vi "Configure Math Basic.vi"(0 "VISA resource name":refnum<visa-resource-name>, 1 "GX/GP START/STOP Key Action (1: Start/Stop)":u16(ring)=1 items=["Off", "Start/Stop", "Reset + Start/Stop"], 5 "Value On Error (0: +Over)":u16(ring) items=["+Over", "-Over"], 7 "Overflow Value 1 (1: Skip)":u16(ring)=1 items=["Error", "Skip", "Limit"], 9 "Overflow Value 2 (0: Over)":u16(ring) items=["Over", "Skip"], 11 "error in (no error)":errorcluster, 12 "GM START Key Action (0: Not Change)":u16(ring) items=["Not Change", "Off", "Start", "Reset + Start"], 13 "GM STOP Key Action (0: Not Change)":u16(ring) items=["Not Change", "Off", "Stop"]) -> (4 "VISA resource name out":refnum<visa-resource-name>, 15 "error out":errorcluster)   [LabVIEW 2020, in "Yokogawa GX Series.lvlib"]
doc: "Sets the basic operation of math channels.\n\nCommand: SMathBasic"
uses:
  <instrlib>/Yokogawa GX Series/Yokogawa GX Series.lvlib
panel:
  in  "PSUM overflow handing (0: ROTATE)":u16(ring) items=["ROTATE", "Over"]
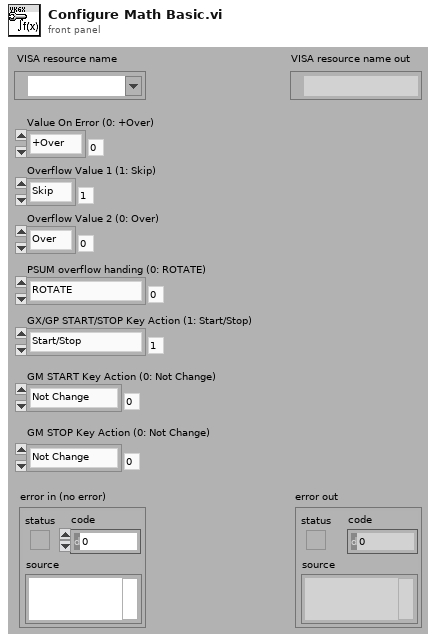
[diagram p1: front panel]
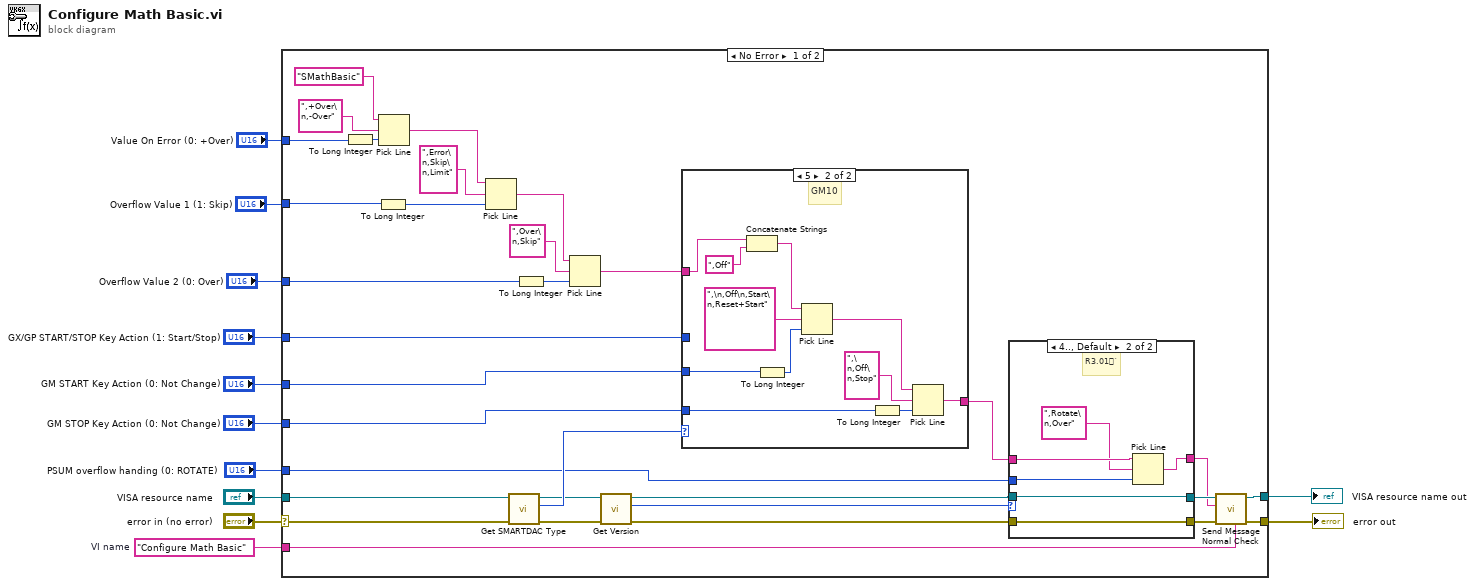
[diagram p0: block diagram]
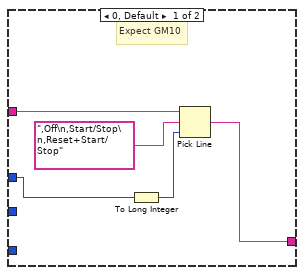
[diagram p3: hidden frame]
diagram:
  w11 = "Configure Math Basic"  # VI name
  n1 = case shown="No Error" "error in (no error)" {
    selector: "error in (no error)" -> [w34 w70]
    tunnel: "VISA resource name" -> [w35 w71]
    tunnel: w11 -> [w44 _]
    tunnel: [w43 w71] -> w10
    tunnel: [w42 w70] -> w9
    tunnel: "Value On Error (0: +Over)" -> [w23 _]
    tunnel: "Overflow Value 1 (1: Skip)" -> [w25 _]
    tunnel: "Overflow Value 2 (0: Over)" -> [w27 _]
    tunnel: "GX/GP START/STOP Key Action (1: Start/Stop)" -> [w31 _]
    tunnel: "GM START Key Action (0: Not Change)" -> [w30 _]
    tunnel: "GM STOP Key Action (0: Not Change)" -> [w29 _]
    tunnel: "PSUM overflow handing (0: ROTATE)" -> [w13 _]
    frame No Error {
      n2 = To Long Integer(number=w23) -> (32bit integer=w24:i32)
      n3 = To Long Integer(number=w25) -> (32bit integer=w26:i32)
      n4 = Pick Line(string ("")="SMathBasic", multi-line string=",+Over\n,-Over", line index=w24) -> (output string=w37:string)
      n5 = Pick Line(string ("")=w37, multi-line string=",Error\n,Skip\n,Limit", line index=w26) -> (output string=w36:string)
      n6 = call <instrlib>:"Get SMARTDAC Type.vi"("error in (no error)"=w34, "VISA resource name"=w35) -> ("error out"=w21:errorcluster, "SMARTDAC+ Type"=w33:u16, "VISA resource name out"=w22:refnum<visa-resource-name>)  [unwired: 7 in]
      n7 = To Long Integer(number=w27) -> (32bit integer=w28:i32)
      n8 = Pick Line(string ("")=w36, multi-line string=",Over\n,Skip", line index=w28) -> (output string=w32:string)
      n9 = call <instrlib>:"Get Version.vi"("error in (no error)"=w21, "VISA resource name"=w22) -> ("error out"=w17:errorcluster, "Version"=w20:i32, "VISA resource name out"=w19:refnum<visa-resource-name>)  [unwired: 7 in]
      n10 = case shown="5" w33 {
        tunnel: w32 -> [w57 w66]
        tunnel: [w56 w63] -> w15
        tunnel: w31 -> [w54 _]
        tunnel: w30 -> [_ w59]
        tunnel: w29 -> [_ w61]
        frame 0, Default {
          # "Expect GM10"
          n11 = To Long Integer(number=w54) -> (32bit integer=w55:i32)
          n12 = Pick Line(string ("")=w57, multi-line string=",Off\n,Start/Stop\n,Reset+Start/Stop", line index=w55) -> (output string=w56:string)
        }
        frame 5 {
          # "GM10"
          n13 = Concatenate Strings(w66, ",Off") -> (w64:string)
          n14 = To Long Integer(number=w59) -> (32bit integer=w60:i32)
          n15 = Pick Line(string ("")=w64, multi-line string=",\n,Off\n,Start\n,Reset+Start", line index=w60) -> (output string=w67:string)
          n16 = To Long Integer(number=w61) -> (32bit integer=w62:i32)
          n17 = Pick Line(string ("")=w67, multi-line string=",\n,Off\n,Stop", line index=w62) -> (output string=w63:string)
        }
      }
      n18 = case shown="4.., Default" w20 {
        tunnel: w19 -> [w47 w53]
        tunnel: [w47 w53] -> w18
        tunnel: w17 -> [w46 w52]
        tunnel: [w46 w52] -> w16
        tunnel: [w45 w50] -> w14
        tunnel: w15 -> [w45 w49]
        tunnel: w13 -> [_ w51]
        frame 0..3 {
          # "R1.03,R2.02,R2.03"
        }
        frame 4.., Default {
          # "R3.01`"
          n19 = Pick Line(string ("")=w49, multi-line string=",Rotate\n,Over", line index=w51) -> (output string=w50:string)
        }
      }
      n20 = call <instrlib>:"Send Message Normal Check.vi"("Source (\"\")"=w44, "error in (no error)"=w16, "Send Message (\"\")"=w14, "VISA resource name"=w18) -> ("error out"=w42:errorcluster, "VISA resource name out"=w43:refnum<visa-resource-name>)  [unwired: 2 in, 4 out]
    }
    frame Error {
    }
  }
  "error out" <- w9
  "VISA resource name out" <- w10
